vi "add vi object.vi"(5 "Ring in":refnum<vi>, 8 "error in (no error)":errorcluster, 10 "Add Object Argument":T1, 11 "Data Cluster in":T2) -> (0 "error out":errorcluster, 1 "Result":string, 2 "object_id":i32, 3 "Data Cluster out":T2)   [LabVIEW 2025, in "Scripting Server.lvlib"]
uses:
  Scripting Server.lvlib
  Module Data--cluster.ctl
  Add Object Argument--cluster.ctl
  Add Object (Reply Payload)--cluster.ctl
  <vilib>/Utility/miscctls.llb/LVPointTypeDef.ctl
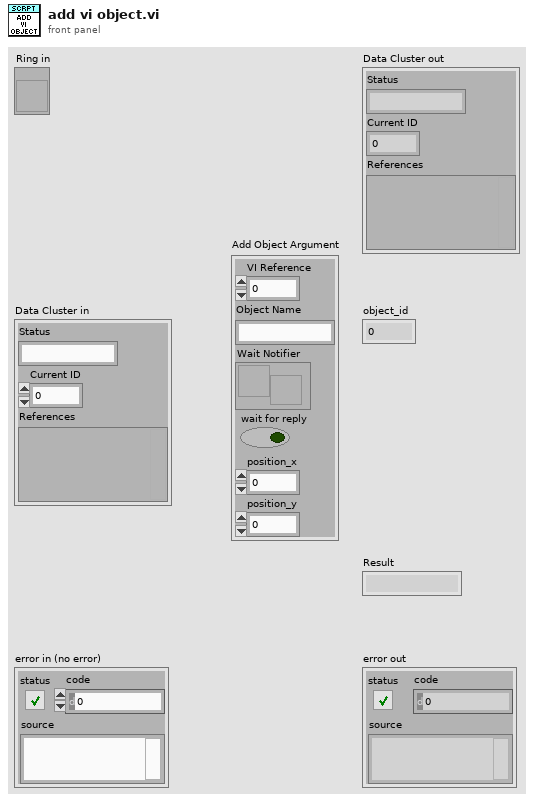
[diagram p1: front panel]
types:
  T1 = typedef "Scripting Server.lvlib/Add Object Argument--cluster.ctl" = cluster{"VI Reference":i32, "Object Name":string, "Wait Notifier":refnum<notifier>, "wait for reply":bool, "position_x":i32, "position_y":i32}
  T2 = typedef "Scripting Server.lvlib/Module Data--cluster.ctl" = cluster{"Status":string, "Current ID":i32, "References":variant}
  T3 = typedef "LVPointTypeDef.ctl" = cluster{"Horizontal":i16, "Vertical":i16}
  T4 = typedef "LVStringsAndValuesArrayTypeDef_I32.ctl" = cluster{"String":string, "Value":i32}[]
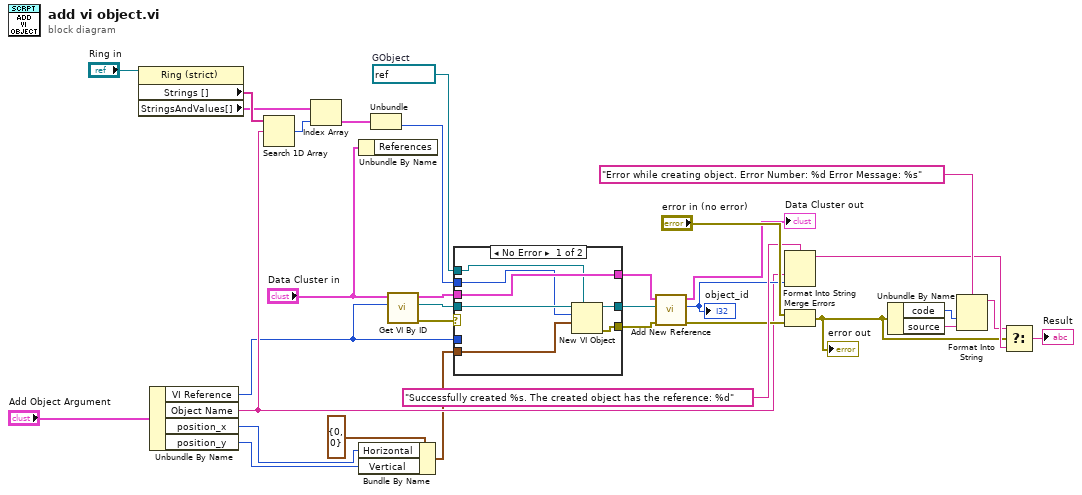
[diagram p0: block diagram]
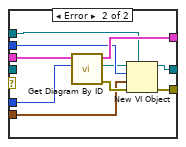
[diagram p2: hidden frame]
diagram:
  w5 = refnum<vi> refnum  # GObject
  n1 = property on="Property Node" class="Ring (strict)"(reference="Ring in") -> ("Strings []"=w31:string[], "StringsAndValues[]"=w30:T4)  [unwired: 1 in, 2 out]
  n2 = Unbundle By Name("Add Object Argument") -> ("VI Reference"=w8:i32, "Object Name"=w12:string, "position_x"=w11:i32, "position_y"=w10:i32)
  n3 = Search 1D Array(1D array=w31, element=w12) -> (index of element=w29:i32)  [unwired: 1 in]
  n4 = Index Array(array=w30, index=w29) -> (element=w32:cluster{"String":string, "Value":i32})
  n5 = Unbundle By Name("Data Cluster in") -> ()  [unwired: 1 out]
  n6 = Bundle By Name(cluster=T3 {"Horizontal"=0, "Vertical"=0} ("location"), "Horizontal"=w11, "Vertical"=w10) -> (w4:T3)
  n7 = Unbundle(w32) -> ("Value"=w3:i32)  [unwired: 1 out]
  n8 = call "Get VI By ID.vi"("ID"=w8, "Data Cluster in"="Data Cluster in") -> ("error out"=w7:errorcluster, "VI Reference"=w6:refnum<vi>, "Data Cluster out"=w9:T2)  [unwired: 7 in]
  n9 = case shown="No Error" w7 {
    tunnel: [w39 w50] -> w14
    tunnel: w8 -> [_ w49]
    tunnel: w9 -> [w39 w48]
    tunnel: w6 -> [w38 _]
    tunnel: w5 -> [w35 w47]
    tunnel: w4 -> [w34 w45]
    tunnel: w3 -> [w36 w44]
    tunnel: [w40 w42] -> w2
    tunnel: [w37 w41] -> w1
    frame No Error {
      n10 = New VI Object(vi object class=w35, owner refnum=w38, style=w36, position/next to=w34) -> (object refnum=w37:refnum<vi>, 0:w40:errorcluster)  [unwired: 4 in]
    }
    frame Error {
      n11 = call "Get Diagram By ID.vi"("ID"=w49, "Data Cluster in"=w48) -> ("error out"=w46:errorcluster, "Diagram"=w43:refnum<vi>, "Data Cluster out"=w50:T2)  [unwired: 7 in]
      n12 = New VI Object(vi object class=w47, owner refnum=w43, style=w44, position/next to=w45, 8:w46) -> (object refnum=w41:refnum<vi>, 0:w42:errorcluster)  [unwired: 3 in]
    }
  }
  n13 = call "Add New Reference.vi"("error in (no error)"=w2, "Variant"=w1, "Data Cluster in"=w14) -> ("error out"=w18:errorcluster, "new reference"=w16:i32, "Data Cluster out 2"=→"Data Cluster out":T2)  [unwired: 6 in]
  "object_id" <- w16
  n14 = Format Into String(format string="Successfully created %s. The created object has the reference: %d", w12, w16) -> (resulting string=w24:string)  [unwired: 2 in, 1 out]
  n15 = Merge Errors("error in (no error)", w18) -> (w21:errorcluster)
  "error out" <- w21
  n16 = Unbundle By Name(w21) -> ("code"=w20:i32, "source"=w19:string)
  n17 = Format Into String(format string="Error while creating object. Error Number: %d Error Message: %s" ("f"), w20, w19) -> (resulting string=w22:string)  [unwired: 2 in, 1 out]
  n18 = Select(t=w22, s=w21, f=w24) -> (s? t:f=→"Result":string)
